vi "range.vi"(4 "felso":dbl=10.0, 6 "also":dbl=0.4, 8 "n":dbl) -> (0 "n2":dbl)   [LabVIEW 2012]
panel:
  out "v":bool
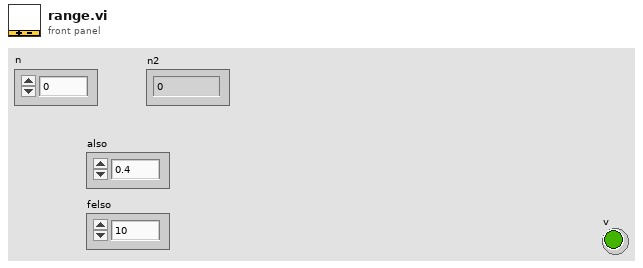
[diagram p1: front panel]
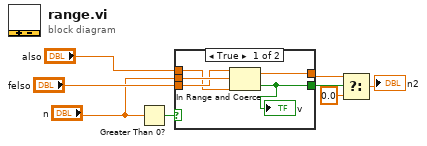
[diagram p0: block diagram]
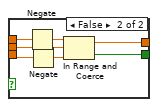
[diagram p2: hidden frame]
diagram:
  n1 = Greater Than 0?(x="n") -> (x > 0?=w8:bool)
  n2 = case shown="True" w8 {
    tunnel: "n" -> [w13 w20]
    tunnel: "felso" -> [w10 w16]
    tunnel: "also" -> [w9 w18]
    tunnel: [w12 w15] -> w3
    tunnel: [w11 w14] -> w5
    frame True {
      n3 = In Range and Coerce(upper limit=w10, x=w13, lower limit=w9) -> (coerced(x)=w12:dbl, In Range?=w11:bool)
      "v" <- w11
    }
    frame False {
      n4 = Negate(x=w18) -> (-x=w19:dbl)
      n5 = Negate(x=w16) -> (-x=w17:dbl)
      n6 = In Range and Coerce(upper limit=w19, x=w20, lower limit=w17) -> (coerced(x)=w15:dbl, In Range?=w14:bool)
    }
  }
  n7 = Select(t=w3, s=w5, f=0.0) -> (s? t:f=→"n2":dbl)
